vi "Parse Token.vi"(8 "Error In":errorcluster, 10 "Token":refnum<class "Token.lvclass">, 11 "Stack In":refnum<queue>) -> (0 "Error Out":errorcluster, 3 "Stack Out":refnum<queue>)   [LabVIEW 2018, in "Toolkit.lvlib" / "Parser.lvclass"]
uses:
  Parser.lvclass
  Nodes/NonTerminal/NonTerminal.lvclass
  D:/Users/cfield/Code/Field R&D Services/Labstache/src/Toolkit/Low-Level/Nodes/Node/Node.lvclass
  Tokens/Token/Token.lvclass
  Tokens/Comment/Comment.lvclass
  Tokens/SetDelimiter/SetDelimiter.lvclass
  Tokens/SetDelimiter/SetDelimiter.lvclass/SetDelimiter.ctl
  Tokens/Text/Text.lvclass
  Nodes/Section/Section.lvclass
  D:/Users/cfield/Code/Field R&D Services/Labstache/src/Toolkit/Low-Level/Nodes/NonTerminal/NonTerminal.lvclass
  Nodes/Comment/Comment.lvclass
  Nodes/Variable/Variable.lvclass
  Nodes/Partial/Partial.lvclass
  Nodes/Delimiter/Delimiter.lvclass
  Nodes/Text/Text.lvclass
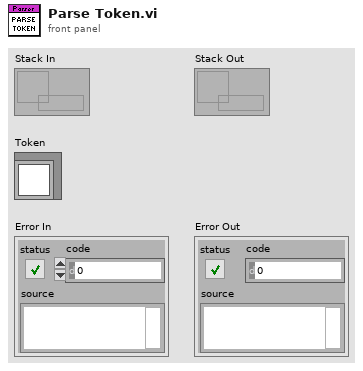
[diagram p1: front panel]
types:
  T1 = typedef "Toolkit.lvlib/Tokens.lvlib/Types.ctl" = enum16{"Begin Section", "Comment", "End Section", "Escaped Variable", "Inverted Section", "Partial", "Set Delimiter", "Text", "Unescaped Variable", "Unknown"}
  T2 = typedef "Toolkit.lvlib/Delimiters.ctl" = cluster{"Close":string, "Open":string}
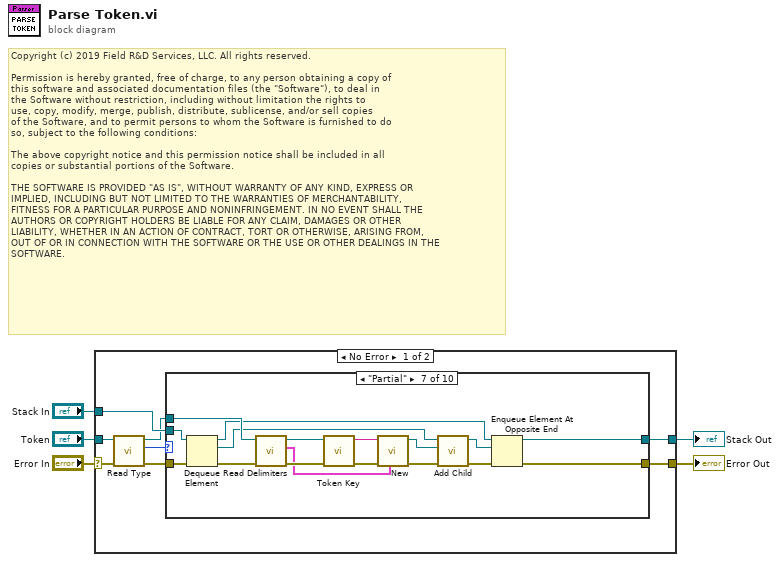
[diagram p0: block diagram]
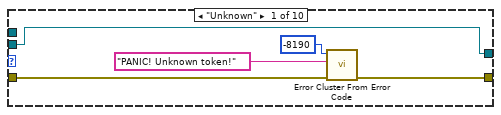
[diagram p2: hidden frame]
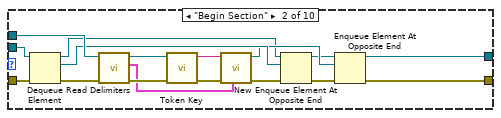
[diagram p3: hidden frame]
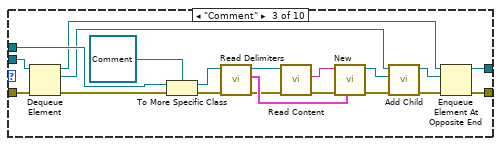
[diagram p4: hidden frame]
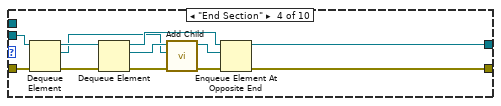
[diagram p5: hidden frame]
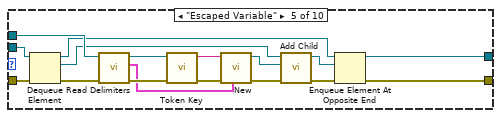
[diagram p6: hidden frame]
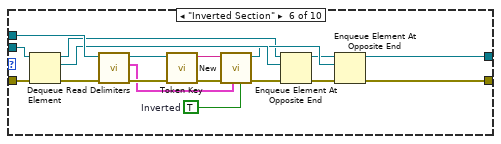
[diagram p7: hidden frame]
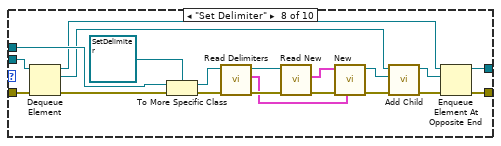
[diagram p8: hidden frame]
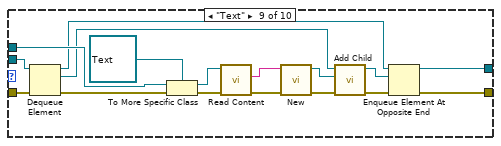
[diagram p9: hidden frame]
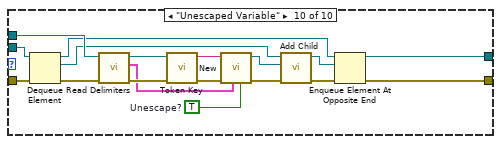
[diagram p10: hidden frame]
diagram:
  # "Copyright (c) 2019 Field R&D Services, LLC. All rights reserved.\n\nPermission is hereby granted, free of charge, to any person obtaining a copy of\nthis software and associated documentation files (the \"Software\"), to deal in\nthe Software without restriction, including without limitation the rights to\nuse, copy, modify, merge, publish, distribute, sublicense, and/or sell copies\nof the Software, and to permit persons to whom the Software is furnished to do\nso, subject to the following conditions:\n\nThe above copyright notice and this permission notice shall be included in all\ncopies or substantial portions of the Software.\n\nTHE SOFTWARE IS PROVIDED \"AS IS\", WITHOUT WARRANTY OF ANY KIND, EXPRESS OR\nIMPLIED, INCLUDING BUT NOT LIMITED TO THE WARRANTIES OF MERCHANTABILITY,\nFITNESS FOR A PARTICULAR PURPOSE AND NONINFRINGEMENT. IN NO EVENT SHALL THE\nAUTHORS OR COPYRIGHT HOLDERS BE LIABLE FOR ANY CLAIM, DAMAGES OR OTHER\nLIABILITY, WHETHER IN AN ACTION OF CONTRACT, TORT OR OTHERWISE, ARISING FROM,\nOUT OF OR IN CONNECTION WITH THE SOFTWARE OR THE USE OR OTHER DEALINGS IN THE\nSOFTWARE."
  n1 = case shown="No Error" "Error In" {
    selector: "Error In" -> [w8 w175]
    tunnel: [w13 w176] -> w5
    tunnel: "Token" -> [w10 _]
    tunnel: [w12 w175] -> w3
    tunnel: "Stack In" -> [w11 w176]
    frame No Error {
      n2 = call-dynamic "Read Type.vi"("Error In"=w8, "Token In"=w10) -> ("Error Out"=w6:errorcluster, "Type"=w7:T1, "Token Out"=w9:refnum<class "Token.lvclass">)  [unwired: 7 in]
      n3 = case shown="\"Partial\"" w7 {
        tunnel: w6 -> [w18 w32 w55 w67 w84 w99 w117 w139 w156 w172]
        tunnel: [w16 w30 w45 w57 w74 w97 w115 w130 w145 w163] -> w12
        tunnel: w9 -> [_ w35 w54 _ w83 w102 w119 w138 w154 w171]
        tunnel: w11 -> [w14 w33 w51 w66 w80 w100 w118 w136 w151 w169]
        tunnel: [w14 w29 w48 w59 w77 w96 w116 w133 w148 w166] -> w13
        frame "Unknown" {
          n4 = call <vilib>:"Error Cluster From Error Code.vi"("error in (no error)"=w18, "error message (\"\")"="PANIC! Unknown token!" ("error message (\"\")"), "error code (0)"=-8190) -> ("error out"=w16:errorcluster)  [unwired: 6 in]
        }
        frame "Begin Section" {
          n5 = Dequeue Element(queue=w33, error in (no error)=w32) -> (queue out=w27:refnum<queue>, element=w31:refnum<class "NonTerminal.lvclass">, error out=w21:errorcluster)  [unwired: 1 in, 1 out]
          n6 = call-dynamic "Read Delimiters.vi"("Error In"=w21, "Token In"=w35) -> ("Error Out"=w20:errorcluster, "Delimiters"=w19:T2, "Token Out"=w22:refnum<class "Token.lvclass">)  [unwired: 7 in]
          n7 = call "Token Key.vi"("Error In"=w20, "Token"=w22) -> ("Error Out"=w24:errorcluster, "Key"=w34:string)  [unwired: 8 in]
          n8 = call "New.vi"("Delimiters"=w19, "Error In"=w24, "Key"=w34) -> ("Error Out"=w23:errorcluster, "Section"=w28:refnum<class "Section.lvclass">)  [unwired: 7 in]
          n9 = Enqueue Element At Opposite End(queue=w27, element=w31, error in (no error)=w23) -> (queue out=w26:refnum<queue>, error out=w25:errorcluster)  [unwired: 1 in, 1 out]
          n10 = Enqueue Element At Opposite End(queue=w26, element=w28, error in (no error)=w25) -> (queue out=w29:refnum<queue>, error out=w30:errorcluster)  [unwired: 1 in, 1 out]
        }
        frame "Comment" {
          n11 = Dequeue Element(queue=w51, error in (no error)=w55) -> (queue out=w49:refnum<queue>, element=w50:refnum<class "NonTerminal.lvclass">, error out=w52:errorcluster)  [unwired: 1 in, 1 out]
          n12 = To More Specific Class(target class=refnum<class "Comment.lvclass"> refnum ("Toolkit.lvlib:Tokens.lvlib:Comment.lvclass"), reference=w54, error in=w52) -> (specific class reference=w40:refnum<class "Comment.lvclass">, error out=w36:errorcluster)
          n13 = call-dynamic "Read Delimiters.vi"("Error In"=w36, "Token In"=w40) -> ("Error Out"=w37:errorcluster, "Delimiters"=w41:T2, "Token Out"=w39:refnum<class "Comment.lvclass">)  [unwired: 7 in]
          n14 = call-dynamic "Read Content.vi"("Error In"=w37, "Contentable In"=w39) -> ("Error Out"=w38:errorcluster, "Content"=w42:string)  [unwired: 7 in, 1 out]
          n15 = call "New.vi"("Delimiters"=w41, "Error In"=w38, "Content"=w42) -> ("Error Out"=w43:errorcluster, "Comment"=w53:refnum<class "Comment.lvclass">)  [unwired: 7 in]
          n16 = call-dynamic "Add Child.vi"("Error In"=w43, "Child"=w53, "Non-Terminal In"=w50) -> ("Error Out"=w46:errorcluster, "Non-Terminal Out"=w47:refnum<class "NonTerminal.lvclass">)  [unwired: 7 in]
          n17 = Enqueue Element At Opposite End(queue=w49, element=w47, error in (no error)=w46) -> (queue out=w48:refnum<queue>, error out=w45:errorcluster)  [unwired: 1 in, 1 out]
        }
        frame "End Section" {
          n18 = Dequeue Element(queue=w66, error in (no error)=w67) -> (queue out=w65:refnum<queue>, element=w61:refnum<class "NonTerminal.lvclass">, error out=w63:errorcluster)  [unwired: 1 in, 1 out]
          n19 = Dequeue Element(queue=w65, error in (no error)=w63) -> (queue out=w64:refnum<queue>, element=w62:refnum<class "NonTerminal.lvclass">, error out=w60:errorcluster)  [unwired: 1 in, 1 out]
          n20 = call-dynamic "Add Child.vi"("Error In"=w60, "Child"=w61, "Non-Terminal In"=w62) -> ("Error Out"=w58:errorcluster, "Non-Terminal Out"=w56:refnum<class "NonTerminal.lvclass">)  [unwired: 7 in]
          n21 = Enqueue Element At Opposite End(queue=w64, element=w56, error in (no error)=w58) -> (queue out=w59:refnum<queue>, error out=w57:errorcluster)  [unwired: 1 in, 1 out]
        }
        frame "Escaped Variable" {
          n22 = Dequeue Element(queue=w80, error in (no error)=w84) -> (queue out=w78:refnum<queue>, element=w79:refnum<class "NonTerminal.lvclass">, error out=w70:errorcluster)  [unwired: 1 in, 1 out]
          n23 = call-dynamic "Read Delimiters.vi"("Error In"=w70, "Token In"=w83) -> ("Error Out"=w69:errorcluster, "Delimiters"=w68:T2, "Token Out"=w71:refnum<class "Token.lvclass">)  [unwired: 7 in]
          n24 = call "Token Key.vi"("Error In"=w69, "Token"=w71) -> ("Error Out"=w73:errorcluster, "Key"=w81:string)  [unwired: 8 in]
          n25 = call "New.vi"("Delimiters"=w68, "Error In"=w73, "Key"=w81) -> ("Error Out"=w72:errorcluster, "Variable"=w82:refnum<class "Variable.lvclass">)  [unwired: 7 in]
          n26 = call-dynamic "Add Child.vi"("Error In"=w72, "Child"=w82, "Non-Terminal In"=w79) -> ("Error Out"=w75:errorcluster, "Non-Terminal Out"=w76:refnum<class "NonTerminal.lvclass">)  [unwired: 7 in]
          n27 = Enqueue Element At Opposite End(queue=w78, element=w76, error in (no error)=w75) -> (queue out=w77:refnum<queue>, error out=w74:errorcluster)  [unwired: 1 in, 1 out]
        }
        frame "Inverted Section" {
          w91 = TRUE  # Inverted
          n28 = Dequeue Element(queue=w100, error in (no error)=w99) -> (queue out=w94:refnum<queue>, element=w98:refnum<class "NonTerminal.lvclass">, error out=w87:errorcluster)  [unwired: 1 in, 1 out]
          n29 = call-dynamic "Read Delimiters.vi"("Error In"=w87, "Token In"=w102) -> ("Error Out"=w86:errorcluster, "Delimiters"=w85:T2, "Token Out"=w88:refnum<class "Token.lvclass">)  [unwired: 7 in]
          n30 = call "Token Key.vi"("Error In"=w86, "Token"=w88) -> ("Error Out"=w90:errorcluster, "Key"=w101:string)  [unwired: 8 in]
          n31 = call "New.vi"("Inverted"=w91, "Delimiters"=w85, "Error In"=w90, "Key"=w101) -> ("Error Out"=w89:errorcluster, "Section"=w95:refnum<class "Section.lvclass">)  [unwired: 6 in]
          n32 = Enqueue Element At Opposite End(queue=w94, element=w98, error in (no error)=w89) -> (queue out=w93:refnum<queue>, error out=w92:errorcluster)  [unwired: 1 in, 1 out]
          n33 = Enqueue Element At Opposite End(queue=w93, element=w95, error in (no error)=w92) -> (queue out=w96:refnum<queue>, error out=w97:errorcluster)  [unwired: 1 in, 1 out]
        }
        frame "Partial" {
          n34 = Dequeue Element(queue=w118, error in (no error)=w117) -> (queue out=w114:refnum<queue>, element=w107:refnum<class "NonTerminal.lvclass">, error out=w112:errorcluster)  [unwired: 1 in, 1 out]
          n35 = call-dynamic "Read Delimiters.vi"("Error In"=w112, "Token In"=w119) -> ("Error Out"=w111:errorcluster, "Delimiters"=w110:T2, "Token Out"=w113:refnum<class "Token.lvclass">)  [unwired: 7 in]
          n36 = call "Token Key.vi"("Error In"=w111, "Token"=w113) -> ("Error Out"=w108:errorcluster, "Key"=w109:string)  [unwired: 8 in]
          n37 = call "New.vi"("Delimiters"=w110, "Error In"=w108, "Key"=w109) -> ("Error Out"=w105:errorcluster, "Partial"=w103:refnum<class "Partial.lvclass">)  [unwired: 7 in]
          n38 = call-dynamic "Add Child.vi"("Error In"=w105, "Child"=w103, "Non-Terminal In"=w107) -> ("Error Out"=w104:errorcluster, "Non-Terminal Out"=w106:refnum<class "NonTerminal.lvclass">)  [unwired: 7 in]
          n39 = Enqueue Element At Opposite End(queue=w114, element=w106, error in (no error)=w104) -> (queue out=w116:refnum<queue>, error out=w115:errorcluster)  [unwired: 1 in, 1 out]
        }
        frame "Set Delimiter" {
          n40 = Dequeue Element(queue=w136, error in (no error)=w139) -> (queue out=w134:refnum<queue>, element=w135:refnum<class "NonTerminal.lvclass">, error out=w137:errorcluster)  [unwired: 1 in, 1 out]
          n41 = To More Specific Class(target class=refnum<class "SetDelimiter.lvclass"> refnum ("Toolkit.lvlib:Tokens.lvlib:SetDelimiter.lvclass"), reference=w138, error in=w137) -> (specific class reference=w129:refnum<class "SetDelimiter.lvclass">, error out=w128:errorcluster)
          n42 = call-dynamic "Read Delimiters.vi"("Error In"=w128, "Token In"=w129) -> ("Error Out"=w126:errorcluster, "Delimiters"=w120:T2, "Token Out"=w125:refnum<class "SetDelimiter.lvclass">)  [unwired: 7 in]
          n43 = call "Read New.vi"("Error In"=w126, "Set Delimiter In"=w125) -> ("Error Out"=w124:errorcluster, "New Value"=w121:cluster{"Close":string, "Open":string})  [unwired: 7 in, 1 out]
          n44 = call "New.vi"("Delimiters"=w120, "Error In"=w124, "New Delimiters"=w121) -> ("Error Out"=w123:errorcluster, "Delimiter"=w122:refnum<class "Delimiter.lvclass">)  [unwired: 7 in]
          n45 = call-dynamic "Add Child.vi"("Error In"=w123, "Child"=w122, "Non-Terminal In"=w135) -> ("Error Out"=w131:errorcluster, "Non-Terminal Out"=w132:refnum<class "NonTerminal.lvclass">)  [unwired: 7 in]
          n46 = Enqueue Element At Opposite End(queue=w134, element=w132, error in (no error)=w131) -> (queue out=w133:refnum<queue>, error out=w130:errorcluster)  [unwired: 1 in, 1 out]
        }
        frame "Text" {
          n47 = Dequeue Element(queue=w151, error in (no error)=w156) -> (queue out=w149:refnum<queue>, element=w150:refnum<class "NonTerminal.lvclass">, error out=w152:errorcluster)  [unwired: 1 in, 1 out]
          n48 = To More Specific Class(target class=refnum<class "Text.lvclass"> refnum ("Toolkit.lvlib:Tokens.lvlib:Text.lvclass"), reference=w154, error in=w152) -> (specific class reference=w143:refnum<class "Text.lvclass">, error out=w142:errorcluster)
          n49 = call-dynamic "Read Content.vi"("Error In"=w142, "Contentable In"=w143) -> ("Error Out"=w140:errorcluster, "Content"=w141:string)  [unwired: 7 in, 1 out]
          n50 = call "New.vi"("Error In"=w140, "Content"=w141) -> ("Error Out"=w144:errorcluster, "Text"=w153:refnum<class "Text.lvclass">)  [unwired: 8 in]
          n51 = call-dynamic "Add Child.vi"("Error In"=w144, "Child"=w153, "Non-Terminal In"=w150) -> ("Error Out"=w146:errorcluster, "Non-Terminal Out"=w147:refnum<class "NonTerminal.lvclass">)  [unwired: 7 in]
          n52 = Enqueue Element At Opposite End(queue=w149, element=w147, error in (no error)=w146) -> (queue out=w148:refnum<queue>, error out=w145:errorcluster)  [unwired: 1 in, 1 out]
        }
        frame "Unescaped Variable" {
          w173 = TRUE  # Unescape?
          n53 = Dequeue Element(queue=w169, error in (no error)=w172) -> (queue out=w167:refnum<queue>, element=w168:refnum<class "NonTerminal.lvclass">, error out=w159:errorcluster)  [unwired: 1 in, 1 out]
          n54 = call-dynamic "Read Delimiters.vi"("Error In"=w159, "Token In"=w171) -> ("Error Out"=w158:errorcluster, "Delimiters"=w157:T2, "Token Out"=w160:refnum<class "Token.lvclass">)  [unwired: 7 in]
          n55 = call "Token Key.vi"("Error In"=w158, "Token"=w160) -> ("Error Out"=w162:errorcluster, "Key"=w170:string)  [unwired: 8 in]
          n56 = call "New.vi"("Unescaped"=w173, "Delimiters"=w157, "Error In"=w162, "Key"=w170) -> ("Error Out"=w161:errorcluster, "Variable"=w174:refnum<class "Variable.lvclass">)  [unwired: 6 in]
          n57 = call-dynamic "Add Child.vi"("Error In"=w161, "Child"=w174, "Non-Terminal In"=w168) -> ("Error Out"=w164:errorcluster, "Non-Terminal Out"=w165:refnum<class "NonTerminal.lvclass">)  [unwired: 7 in]
          n58 = Enqueue Element At Opposite End(queue=w167, element=w165, error in (no error)=w164) -> (queue out=w166:refnum<queue>, error out=w163:errorcluster)  [unwired: 1 in, 1 out]
        }
      }
    }
    frame Error {
    }
  }
  "Stack Out" <- w5
  "Error Out" <- w3
